vi "readClientID.vi"(8 "error in (no error)":errorcluster, 11 "MQTTclient in":refnum<class "MQTTclient.lvclass">) -> (0 "error out":errorcluster, 2 "ClientId":string, 3 "MQTTclient out":refnum<class "MQTTclient.lvclass">)   [LabVIEW 2017, in "MQTTclient.lvclass"]
uses:
  MQTTclient.lvclass
  MQTTclient.lvclass/MQTTclient.ctl
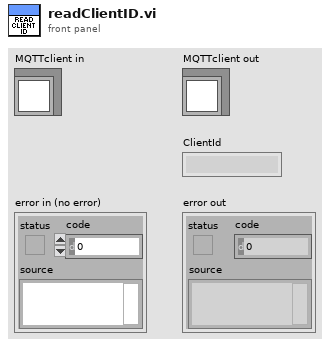
[diagram p1: front panel]
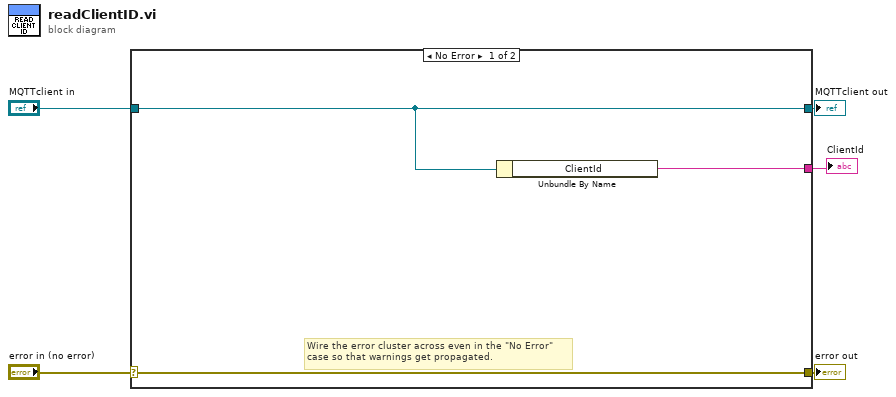
[diagram p0: block diagram]
diagram:
  n1 = case shown="No Error" "error in (no error)" {
    selector: "error in (no error)" -> [w8 w10]
    tunnel: [w8 w10] -> w4
    tunnel: [w7 w9] -> w2
    tunnel: "MQTTclient in" -> [w7 w9]
    tunnel: [w6 _] -> w1
    frame No Error {
      # "Wire the error cluster across even in the \"No Error\"\ncase so that warnings get propagated."
      n2 = Unbundle By Name(w7) -> ("ClientId"=w6:string)
    }
    frame Error {
    }
  }
  "error out" <- w4
  "MQTTclient out" <- w2
  "ClientId" <- w1
